vi "Create Table Heading.vi"(11 "table name":string) -> (0 "table end":string, 3 "table start":string)   [LabVIEW 2019, in "infolib.lvlib"]
doc: "Create heading and tail for the table."
uses:
  infolib.lvlib
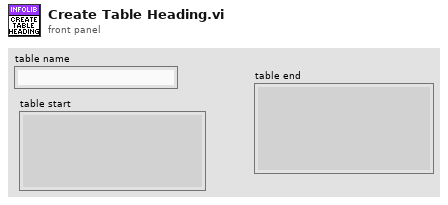
[diagram p1: front panel]
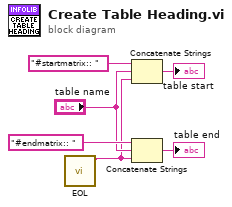
[diagram p0: block diagram]
diagram:
  n1 = call "EOL.vi"() -> ("eol"=w1:string)  [unwired: 11 in]
  n2 = Concatenate Strings("#startmatrix:: " ("string"), "table name", w1) -> (→"table start":string)
  n3 = Concatenate Strings("#endmatrix:: " ("string"), "table name", w1) -> (→"table end":string)
